vi "更新面板列表到树.vi"(10 "pannel-list":T1(array[cluster]), 11 "panel":refnum<vi>) -> ()   [LabVIEW 2019]
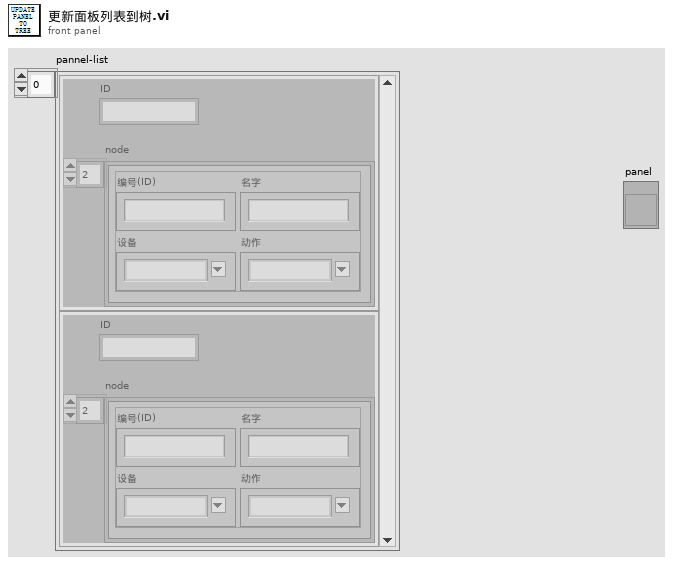
[diagram p1: front panel]
types:
  T1 = cluster{"node":cluster{"ID":string, "Attribute":string, "Action":string, "name":string}[], "ID":string}[]
  T2 = cluster{"ID":string, "Attribute":string, "Action":string, "name":string}[]
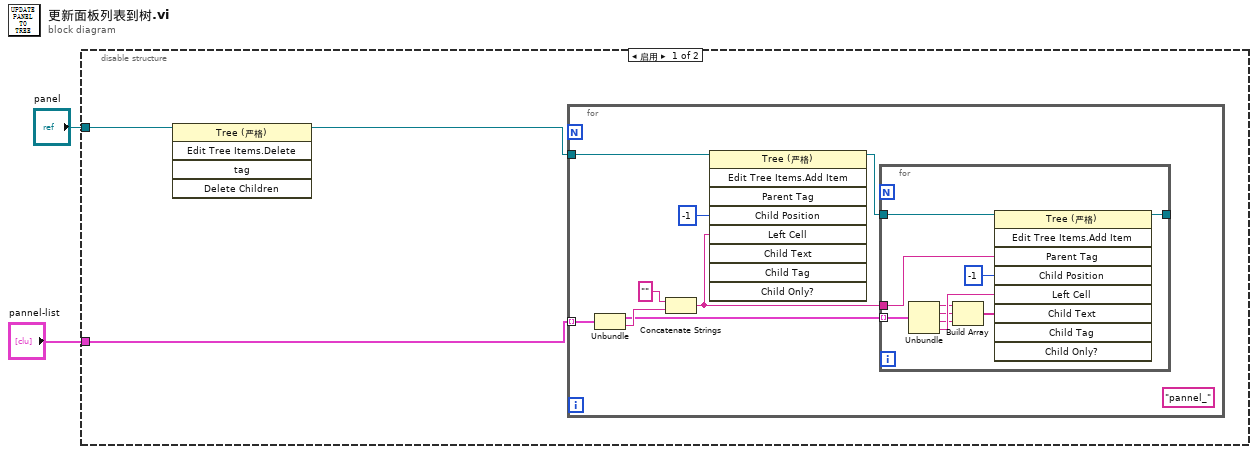
[diagram p0: block diagram]
diagram:
  n1 = disable-structure shown="启用" {
    disable-tunnel: "panel" -> [w4 _]
    disable-tunnel: "pannel-list" -> [w3 _]
    frame Enabled {
      n2 = invoke class="Tree (严格)" method="Edit Tree Items.Delete"(reference=w4) -> (reference out=w5:refnum<vi>)  [unwired: 4 in, 4 out]
      n3 = for {
        tunnel: w3 -> [w13] mode=indexing
        tunnel: w5 -> [w7]
        (unwired) "pannel_" ("字符串")
        n4 = Unbundle(w13) -> ("node"=w10:T2, "ID"=w12:string)
        n5 = Concatenate Strings("" ("字符串"), w12) -> (w9:string)
        n6 = invoke class="Tree (严格)" method="Edit Tree Items.Add Item"(reference=w7, "Child Position"=-1 ("子项位置"), "Left Cell"=w9) -> (reference out=w8:refnum<vi>)  [unwired: 6 in, 8 out]
        n7 = for {
          tunnel: w10 -> [w21] mode=indexing
          tunnel: w8 -> [w23]
          tunnel: w9 -> [w22]
          tunnel: [w19] -> _
          n8 = Unbundle(w21) -> ("ID"=w18:string, "Attribute"=w17:string, "Action"=w16:string, "name"=w20:string)
          n9 = Build Array(w18, w17, w16) -> (w15:string[])
          n10 = invoke class="Tree (严格)" method="Edit Tree Items.Add Item"(reference=w23, "Parent Tag"=w22, "Child Position"=-1 ("子项位置"), "Left Cell"=w20, "Child Text"=w15) -> (reference out=w19:refnum<vi>)  [unwired: 4 in, 8 out]
        }
      }
    }
    frame Disabled {
    }
  }
